vi "Swerve Test.vi"   [LabVIEW 2019]
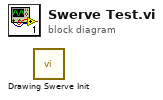
[diagram p0: block diagram]
diagram:
  n1 = call "Drawing Swerve Init.vi"() -> ()  [unwired: 10 in, 2 out]
